vi "linearAnalysis.vi"(7 "deltaPeakTimes":dbl[](array[numeric]) format="%0.2f") -> (4 "meanRR":dbl format="%0.2f", 6 "stdRR":dbl format="%0.2f", 8 "RMSSD":dbl, 10 "NN50":i16, 15 "pNN50":dbl)   [LabVIEW 2025]
uses:
  <vilib>/Analysis/baseanly.llb/Mean (DBL).vi
  <vilib>/Analysis/NI_AALBase.lvlib
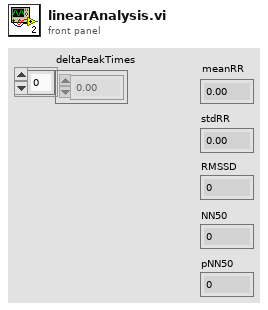
[diagram p1: front panel]
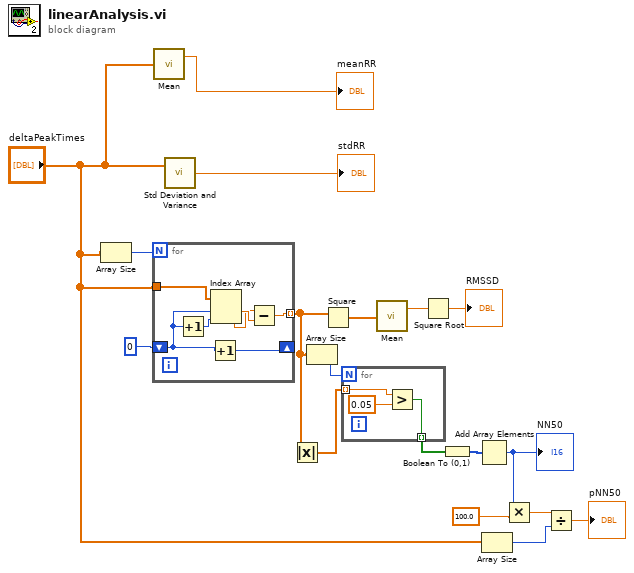
[diagram p0: block diagram]
diagram:
  n1 = Array Size(array="deltaPeakTimes") -> (size(s)=w16:i32)
  n2 = for {
    N: w16 -> [_]
    tunnel: "deltaPeakTimes" -> [w25]
    tunnel: [w23] -> w4 mode=indexing
    shift-right: [w19] -> _
    shift-left: 0 -> [w20]
    n3 = Increment(x=w20) -> (x+1=w24:i32)
    n4 = Increment(x=w20) -> (x+1=w19:i32)
    n5 = Index Array(array=w25, index #1=w20, index #2=w24) -> (element #1=w22:dbl, element #2=w21:dbl)
    n6 = Subtract(x=w21, y=w22) -> (x-y=w23:dbl)
  }
  n7 = call-poly <vilib>:"Mean.vi"("X"="deltaPeakTimes") -> ("mean"=→"meanRR":dbl)  [unwired: 1 out]
  n8 = call <vilib>:"Std Deviation and Variance.vi"("X"="deltaPeakTimes") -> ("standard deviation"=→"stdRR":dbl)  [unwired: 1 in, 2 out]
  n9 = Absolute Value(x=w4) -> (abs(x)=w6:dbl[])
  n10 = Array Size(array=w4) -> (size(s)=w5:i32)
  n11 = Square(x=w4) -> (x^2=w7:dbl[])
  n12 = for {
    N: w5 -> [_]
    tunnel: w6 -> [w27] mode=indexing
    tunnel: [w26] -> w3 mode=indexing
    n13 = Greater?(x=w27, y=0.05) -> (0:w26:bool)
  }
  n14 = call-poly <vilib>:"Mean.vi"("X"=w7) -> ("mean"=w15:dbl)  [unwired: 1 out]
  n15 = Square Root(x=w15) -> (sqrt(x)=→"RMSSD":dbl)
  n16 = Boolean To (0,1)(Boolean=w3) -> (0, 1=w13:i16[])
  n17 = Add Array Elements(numeric array=w13) -> (sum=w11:i16)
  "NN50" <- w11
  n18 = Array Size(array="deltaPeakTimes") -> (size(s)=w9:i32)
  n19 = Multiply(x=w11, y=100.0 ("x")) -> (x*y=w10:dbl)
  n20 = Divide(x=w10, y=w9) -> (x/y=→"pNN50":dbl)
